vi "rsidr_core_global.vi"() -> ()   [LabVIEW 2020, in "Rohde&Schwarz RTx Oscilloscopes.lvlib"] (continued)
"Descriptive Name"="Start Power Safe Operating Area Measurement", "Data Type"=4, "Command"="POW:SOA:EXEC", "Access"=1, "Range Table"="", "Read Callback"="", "Write Callback"="", "Supported Models"="RTM|RTA", "Instrument Options"="", "Flags"=0, "Help"="Starts the safe operating area measurement.\n\nAvailable Repeated Capabilities:\nNone\n\nRemote-control command(s):\nPOWer:SOA:EXECute"}, {"Level"=3, "Class Only"=FALSE, "Identifier"="RSRTX_ATTR_RESTART_POWER_SAFE_OPERATING_AREA_MEASUREMENT", "Descriptive Name"="Restart Power Safe Operating Area Measurement", "Data Type"=4, "Command"="POW:SOA:REST", "Access"=1, "Range Table"="", "Read Callback"="", "Write Callback"="", "Supported Models"="RTM|RTA", "Instrument Options"="", "Flags"=0, "Help"="Restarts the measurement.\n\nAvailable Repeated Capabilities:\nNone\n\nRemote-control command(s):\nPOWer:SOA:RESTart"}, {"Level"=3, "Class Only"=FALSE, "Identifier"="RSRTX_ATTR_POWER_SAFE_OPERATING_AREA_ADD_REPORT", "Descriptive Name"="Power Safe Operating Area Add Report", "Data Type"=4, "Command"="POW:SOA:REP:ADD", "Access"=1, "Range Table"="", "Read Callback"="", "Write Callback"="", "Supported Models"="RTM|RTA", "Instrument Options"="", "Flags"=1, "Help"="Adds the result to the report list.\n\nAvailable Repeated Capabilities:\nNone\n\nRemote-control command(s):\nPOWer:SOA:REPort:ADD"}, {"Level"=3, "Class Only"=FALSE, "Identifier"="RSRTX_ATTR_POWER_SAFE_OPERATING_AREA_SCALE", "Descriptive Name"="Power Safe Operating Area Scale", "Data Type"=0, "Command"="POW:SOA:SCAL", "Access"=2, "Range Table"="rsrtx_rngScaleLinLog", "Read Callback"="", "Write Callback"="", "Supported Models"="RTM|RTA", "Instrument Options"="", "Flags"=0, "Help"="Sets the scale for the measurement.\n\nAvailable Repeated Capabilities:\nNone\n\nRemote-control command(s):\nPOWer:SOA:SCALe"}, {"Level"=3, "Class Only"=FALSE, "Identifier"="RSRTX_ATTR_POWER_SAFE_OPERATING_AREA_MASK_SCALE", "Descriptive Name"="Power Safe Operating Area Mask Scale", "Data Type"=0, "Command"="POW:SOA:SCAL:MASK", "Access"=2, "Range Table"="rsrtx_rngScaleLinLog", "Read Callback"="", "Write Callback"="", "Supported Models"="RTM|RTA", "Instrument Options"="", "Flags"=0, "Help"="Sets the scale for the mask, linear or logarithmic.\n\nAvailable Repeated Capabilities:\nNone\n\nRemote-control command(s):\nPOWer:SOA:SCALe:MASK"}, {"Level"=3, "Class Only"=FALSE, "Identifier"="RSRTX_ATTR_POWER_SAFE_OPERATING_AREA_DISPLAY_SCALE", "Descriptive Name"="Power Safe Operating Area Display Scale", "Data Type"=0, "Command"="POW:SOA:SCAL:DISP", "Access"=2, "Range Table"="rsrtx_rngScaleLinLog", "Read Callback"="", "Write Callback"="", "Supported Models"="RTM|RTA", "Instrument Options"="", "Flags"=0, "Help"="Sets a linear or a logarithmic scaled for the displayed results.\n\nAvailable Repeated Capabilities:\nNone\n\nRemote-control command(s):\nPOWer:SOA:SCALe:DISPlay"}, {"Level"=3, "Class Only"=FALSE, "Identifier"="RSRTX_ATTR_POWER_SAFE_OPERATING_AREA_LIN_ADD", "Descriptive Name"="Power Safe Operating Area Linear Add", "Data Type"=4, "Command"="POW:SOA:LIN:ADD", "Access"=1, "Range Table"="", "Read Callback"="", "Write Callback"="", "Supported Models"="RTM|RTA", "Instrument Options"="", "Flags"=0, "Help"="Adds a point.\n\nAvailable Repeated Capabilities:\nNone\n\nRemote-control command(s):\nPOWer:SOA:LINear:ADD"}, {"Level"=3, "Class Only"=FALSE, "Identifier"="RSRTX_ATTR_POWER_SAFE_OPERATING_AREA_LINEAR_INSERT", "Descriptive Name"="Power Safe Operating Area Linear Insert", "Data Type"=0, "Command"="POW:SOA:LIN:INS", "Access"=1, "Range Table"="", "Read Callback"="", "Write Callback"="", "Supported Models"="RTM|RTA", "Instrument Options"="", "Flags"=0, "Help"="Inserts a point.\n\nAvailable Repeated Capabilities:\nNone\n\nRemote-control command(s):\nPOWer:SOA:LINear:INSert"}, {"Level"=3, "Class Only"=FALSE, "Identifier"="RSRTX_ATTR_POWER_SAFE_OPERATING_AREA_LINEAR_REMOVE", "Descriptive Name"="Power Safe Operating Area Linear Remove", "Data Type"=0, "Command"="POW:SOA:LIN:REM", "Access"=1, "Range Table"="", "Read Callback"="", "Write Callback"="", "Supported Models"="RTM|RTA", "Instrument Options"="", "Flags"=0, "Help"="Removes a point.\n\nAvailable Repeated Capabilities:\nNone\n\nRemote-control command(s):\nPOWer:SOA:LINear:REMove"}, {"Level"=3, "Class Only"=FALSE, "Identifier"="RSRTX_ATTR_POWER_SAFE_OPERATING_AREA_LINEAR_COUNT", "Descriptive Name"="Power Safe Operating Area Linear Count", "Data Type"=0, "Command"="POW:SOA:LIN:COUN?", "Access"=0, "Range Table"="", "Read Callback"="", "Write Callback"="", "Supported Models"="RTM|RTA", "Instrument Options"="", "Flags"=0, "Help"="Queries the number of points.\n\nAvailable Repeated Capabilities:\nNone\n\nRemote-control command(s):\nPOWer:SOA:LINear:COUNt?"}, {"Level"=3, "Class Only"=FALSE, "Identifier"="RSRTX_ATTR_POWER_SAFE_OPERATING_AREA_LOGARITHMIC_ADD", "Descriptive Name"="Power Safe Operating Area Logarithmic Add", "Data Type"=4, "Command"="POW:SOA:LOG:ADD", "Access"=1, "Range Table"="", "Read Callback"="", "Write Callback"="", "Supported Models"="RTM|RTA", "Instrument Options"="", "Flags"=0, "Help"="Adds a point.\n\nAvailable Repeated Capabilities:\nNone\n\nRemote-control command(s):\nPOWer:SOA:LOGarithmic:ADD"}, {"Level"=3, "Class Only"=FALSE, "Identifier"="RSRTX_ATTR_POWER_SAFE_OPERATING_AREA_LOGARITHMIC_INSERT", "Descriptive Name"="Power Safe Operating Area Logarithmic Insert", "Data Type"=0, "Command"="POW:SOA:LOG:INS", "Access"=1, "Range Table"="", "Read Callback"="", "Write Callback"="", "Supported Models"="RTM|RTA", "Instrument Options"="", "Flags"=0, "Help"="Inserts a point.\n\nAvailable Repeated Capabilities:\nNone\n\nRemote-control command(s):\nPOWer:SOA:LOGarithmic:INSert"}, {"Level"=3, "Class Only"=FALSE, "Identifier"="RSRTX_ATTR_POWER_SAFE_OPERATING_AREA_LOGARITHMIC_REMOVE", "Descriptive Name"="Power Safe Operating Area Logarithmic Remove", "Data Type"=0, "Command"="POW:SOA:LOG:REM", "Access"=1, "Range Table"="", "Read Callback"="", "Write Callback"="", "Supported Models"="RTM|RTA", "Instrument Options"="", "Flags"=0, "Help"="Removes a point.\n\nAvailable Repeated Capabilities:\nNone\n\nRemote-control command(s):\nPOWer:SOA:LOGarithmic:REMove"}, {"Level"=3, "Class Only"=FALSE, "Identifier"="RSRTX_ATTR_POWER_SAFE_OPERATING_AREA_LOGARITHMIC_COUNT", "Descriptive Name"="Power Safe Operating Area Logarithmic Count", "Data Type"=0, "Command"="POW:SOA:LOG:COUN?", "Access"=0, "Range Table"="", "Read Callback"="", "Write Callback"="", "Supported Models"="RTM|RTA", "Instrument Options"="", "Flags"=0, "Help"="Queries the number of points.\n\nAvailable Repeated Capabilities:\nNone\n\nRemote-control command(s):\nPOWer:SOA:LOGarithmic:COUNt?"}, {"Level"=3, "Class Only"=FALSE, "Identifier"="RSRTX_ATTR_POWER_SAFE_OPERATING_AREA_SELECTED_POINT", "Descriptive Name"="Power Safe Operating Area Selected Point", "Data Type"=0, "Command"="", "Access"=2, "Range Table"="", "Read Callback"="", "Write Callback"="", "Supported Models"="", "Instrument Options"="", "Flags"=0, "Help"="Sets selector repeated capability Point.\n\nAvailable Repeated Capabilities:\nNone\n\nRemote-control command(s):\n"}, {"Level"=3, "Class Only"=TRUE, "Identifier"="", "Descriptive Name"="Point", "Data Type"=0, "Command"="", "Access"=0, "Range Table"="", "Read Callback"="", "Write Callback"="", "Supported Models"="", "Instrument Options"="", "Flags"=0, "Help"="Class for Point repcap. Points is selected with attribute RSRTX_ATTR_POWER_SAFE_OPERATING_AREA_SELECTED_POINT."}, {"Level"=4, "Class Only"=FALSE, "Identifier"="RSRTX_ATTR_POWER_SAFE_OPERATING_AREA_LINEAR_POINT_VOLTAGE", "Descriptive Name"="Power Safe Operating Area Linear Point Voltage", "Data Type"=1, "Command"="POW:SOA:LIN:POIN<Point>:VOLT", "Access"=2, "Range Table"="", "Read Callback"="rsrtx_FormatSOAPointRepCapReal_ReadCallback.vi", "Write Callback"="rsrtx_FormatSOAPointRepCapReal_WriteCallback.vi", "Supported Models"="RTM|RTA", "Instrument Options"="", "Flags"=0, "Help"="Sets the voltage for the correponding point.\n\nAvailable Repeated Capabilities:\nNone\n\nRemote-control command(s):\nPOWer:SOA:LINear:POINt<m>:VOLTage"}, {"Level"=4, "Class Only"=FALSE, "Identifier"="RSRTX_ATTR_POWER_SAFE_OPERATING_AREA_LINEAR_POINT_CURRENT", "Descriptive Name"="Power Safe Operating Area Linear Point Current", "Data Type"=1, "Command"="POW:SOA:LIN:POIN<Point>:CURR", "Access"=2, "Range Table"="", "Read Callback"="rsrtx_FormatSOAPointRepCapReal_ReadCallback.vi", "Write Callback"="rsrtx_FormatSOAPointRepCapReal_WriteCallback.vi", "Supported Models"="RTM|RTA", "Instrument Options"="", "Flags"=0, "Help"="Sets the current for the correponding point.\n\nAvailable Repeated Capabilities:\nNone\n\nRemote-control command(s):\nPOWer:SOA:LINear:POINt<m>:CURRent"}, {"Level"=4, "Class Only"=FALSE, "Identifier"="RSRTX_ATTR_POWER_SAFE_OPERATING_AREA_LINEAR_POINT_CURRENT_MIN", "Descriptive Name"="Power Safe Operating Area Linear Point Current Min", "Data Type"=1, "Command"="POW:SOA:LIN:POIN<Point>:CURR:MIN", "Access"=2, "Range Table"="", "Read Callback"="rsrtx_FormatSOAPointRepCapReal_ReadCallback.vi", "Write Callback"="rsrtx_FormatSOAPointRepCapReal_WriteCallback.vi", "Supported Models"="RTM|RTA", "Instrument Options"="", "Flags"=0, "Help"="Sets the minimum current for the correponding point.\n\nAvailable Repeated Capabilities:\nNone\n\nRemote-control command(s):\nPOWer:SOA:LINear:POINt<m>:CURRent:MINimum"}, {"Level"=4, "Class Only"=FALSE, "Identifier"="RSRTX_ATTR_POWER_SAFE_OPERATING_AREA_LINEAR_POINT_CURRENT_MAX", "Descriptive Name"="Power Safe Operating Area Linear Point Current Max", "Data Type"=1, "Command"="POW:SOA:LIN:POIN<Point>:CURR:MAX", "Access"=2, "Range Table"="", "Read Callback"="rsrtx_FormatSOAPointRepCapReal_ReadCallback.vi", "Write Callback"="rsrtx_FormatSOAPointRepCapReal_WriteCallback.vi", "Supported Models"="RTM|RTA", "Instrument Options"="", "Flags"=0, "Help"="Sets the maximum current for the correponding point.\n\nAvailable Repeated Capabilities:\nNone\n\nRemote-control command(s):\nPOWer:SOA:LINear:POINt<m>:CURRent:MAXimum"}, {"Level"=4, "Class Only"=FALSE, "Identifier"="RSRTX_ATTR_POWER_SAFE_OPERATING_AREA_LOGARITHMIC_POINT_VOLTAGE", "Descriptive Name"="Power Safe Operating Area Logarithmic Point Voltage", "Data Type"=1, "Command"="POW:SOA:LOG:POIN<Point>:VOLT", "Access"=2, "Range Table"="", "Read Callback"="rsrtx_FormatSOAPointRepCapReal_ReadCallback.vi", "Write Callback"="rsrtx_FormatSOAPointRepCapReal_WriteCallback.vi", "Supported Models"="RTM|RTA", "Instrument Options"="", "Flags"=0, "Help"="Sets the voltage for the correponding point.\n\nAvailable Repeated Capabilities:\nNone\n\nRemote-control command(s):\nPOWer:SOA:LOGarithmic:POINt<m>:VOLTage"}, {"Level"=4, "Class Only"=FALSE, "Identifier"="RSRTX_ATTR_POWER_SAFE_OPERATING_AREA_LOGARITHMIC_POINT_CURRENT", "Descriptive Name"="Power Safe Operating Area Logarithmic Point Current", "Data Type"=1, "Command"="POW:SOA:LOG:POIN<Point>:CURR", "Access"=2, "Range Table"="", "Read Callback"="rsrtx_FormatSOAPointRepCapReal_ReadCallback.vi", "Write Callback"="rsrtx_FormatSOAPointRepCapReal_WriteCallback.vi", "Supported Models"="RTM|RTA", "Instrument Options"="", "Flags"=0, "Help"="Sets the current for the correponding point.\n\nAvailable Repeated Capabilities:\nNone\n\nRemote-control command(s):\nPOWer:SOA:LOGarithmic:POINt<m>:CURRent"}, {"Level"=4, "Class Only"=FALSE, "Identifier"="RSRTX_ATTR_POWER_SAFE_OPERATING_AREA_LOGARITHMIC_POINT_CURRENT_MIN", "Descriptive Name"="Power Safe Operating Area Logarithmic Point Current Min", "Data Type"=1, "Command"="POW:SOA:LOG:POIN<Point>:CURR:MIN", "Access"=2, "Range Table"="", "Read Callback"="rsrtx_FormatSOAPointRepCapReal_ReadCallback.vi", "Write Callback"="rsrtx_FormatSOAPointRepCapReal_WriteCallback.vi", "Supported Models"="RTM|RTA", "Instrument Options"="", "Flags"=0, "Help"="Sets the minimum current for the correponding point.\n\nAvailable Repeated Capabilities:\nNone\n\nRemote-control command(s):\nPOWer:SOA:LOGarithmic:POINt<m>:CURRent:MINimum"}, {"Level"=4, "Class Only"=FALSE, "Identifier"="RSRTX_ATTR_POWER_SAFE_OPERATING_AREA_LOGARITHMIC_POINT_CURRENT_MAX", "Descriptive Name"="Power Safe Operating Area Logarithmic Point Current Max", "Data Type"=1, "Command"="POW:SOA:LOG:POIN<Point>:CURR:MAX", "Access"=2, "Range Table"="", "Read Callback"="rsrtx_FormatSOAPointRepCapReal_ReadCallback.vi", "Write Callback"="rsrtx_FormatSOAPointRepCapReal_WriteCallback.vi", "Supported Models"="RTM|RTA", "Instrument Options"="", "Flags"=0, "Help"="Sets the maximum current for the correponding point.\n\nAvailable Repeated Capabilities:\nNone\n\nRemote-control command(s):\nPOWer:SOA:LOGarithmic:POINt<m>:CURRent:MAXimum"}, {"Level"=3, "Class Only"=TRUE, "Identifier"="", "Descriptive Name"="Results", "Data Type"=0, "Command"="", "Access"=0, "Range Table"="", "Read Callback"="", "Write Callback"="", "Supported Models"="", "Instrument Options"="", "Flags"=0, "Help"="The results of &quot;Safe Operating Area&quot; measurements."}, {"Level"=4, "Class Only"=TRUE, "Identifier"="", "Descriptive Name"="Acquisition", "Data Type"=0, "Command"="", "Access"=0, "Range Table"="", "Read Callback"="", "Write Callback"="", "Supported Models"="", "Instrument Options"="", "Flags"=0, "Help"="Acquisition results."}, {"Level"=5, "Class Only"=FALSE, "Identifier"="RSRTX_ATTR_POWER_SAFE_OPERATING_AREA_RESULT_ACQUISITION_TOLERANCE", "Descriptive Name"="Power Safe Operating Area Result Acquisition Tolerance", "Data Type"=1, "Command"="POW:SOA:RES:ACQ:TOL", "Access"=2, "Range Table"="", "Read Callback"="", "Write Callback"="", "Supported Models"="RTM|RTA", "Instrument Options"="", "Flags"=0, "Help"="Sets acquisition tolerance in percent.\n\nAvailable Repeated Capabilities:\nNone\n\nRemote-control command(s):\nPOWer:SOA:RESult:ACQuisition:TOLerance"}, {"Level"=5, "Class Only"=FALSE, "Identifier"="RSRTX_ATTR_POWER_SAFE_OPERATING_AREA_RESULT_ACQUISITION_PASSED_RESULTS", "Descriptive Name"="Power Safe Operating Area Result Acquisition Passed Results", "Data Type"=0, "Command"="POW:SOA:RES:ACQ:PASS?", "Access"=0, "Range Table"="", "Read Callback"="", "Write Callback"="", "Supported Models"="RTM|RTA", "Instrument Options"="", "Flags"=0, "Help"="Returns the number of passed points, i.e they are within the defined safe operating area.\n\nAvailable Repeated Capabilities:\nNone\n\nRemote-control command(s):\nPOWer:SOA:RESult:ACQuisition:PASSed?"}, {"Level"=5, "Class Only"=FALSE, "Identifier"="RSRTX_ATTR_POWER_SAFE_OPERATING_AREA_RESULT_ACQUISITION_FAILED_RESULTS", "Descriptive Name"="Power Safe Operating Area Result Acquisition Failed Results", "Data Type"=0, "Command"="POW:SOA:RES:ACQ:FAIL?", "Access"=0, "Range Table"="", "Read Callback"="", "Write Callback"="", "Supported Models"="RTM|RTA", "Instrument Options"="", "Flags"=0, "Help"="Returns the number of points that failed, i.e they are not within the defined safe operating area.\n\nAvailable Repeated Capabilities:\nNone\n\nRemote-control command(s):\nPOWer:SOA:RESult:ACQuisition:FAILed?"}, {"Level"=5, "Class Only"=FALSE, "Identifier"="RSRTX_ATTR_POWER_SAFE_OPERATING_AREA_RESULT_ACQUISITION_FAILED_RATE", "Descriptive Name"="Power Safe Operating Area Result Acquisition Failed Rate", "Data Type"=1, "Command"="POW:SOA:RES:ACQ:FRAT?", "Access"=0, "Range Table"="", "Read Callback"="", "Write Callback"="", "Supported Models"="RTM|RTA", "Instrument Options"="", "Flags"=0, "Help"="Returns the total point fail rate, i.e the ratio of point hits to the number of tested points for the current acquisition.\n\nAvailable Repeated Capabilities:\nNone\n\nRemote-control command(s):\nPOWer:SOA:RESult:ACQuisition:FRATe?"}, {"Level"=5, "Class Only"=FALSE, "Identifier"="RSRTX_ATTR_POWER_SAFE_OPERATING_AREA_RESULT_ACQUISITION_NUMBER_OF_POINTS", "Descriptive Name"="Power Safe Operating Area Result Acquisition Number Of Points", "Data Type"=0, "Command"="POW:SOA:RES:ACQ:POIN?", "Access"=0, "Range Table"="", "Read Callback"="", "Write Callback"="", "Supported Models"="RTM|RTA", "Instrument Options"="", "Flags"=0, "Help"="Returns the number of points, considered for the current acquisition.\n\nAvailable Repeated Capabilities:\nNone\n\nRemote-control command(s):\nPOWer:SOA:RESult:ACQuisition:POINts?"}, {"Level"=5, "Class Only"=FALSE, "Identifier"="RSRTX_ATTR_POWER_SAFE_OPERATING_AREA_RESULT_ACQUISITION_STATUS", "Descriptive Name"="Power Safe Operating Area Result Acquisition Status", "Data Type"=3, "Command"="POW:SOA:RES:ACQ:STAT?", "Access"=0, "Range Table"="", "Read Callback"="", "Write Callback"="", "Supported Models"="RTM|RTA", "Instrument Options"="", "Flags"=0, "Help"="Returns the result, passed or failed, of the current aqcuisition measurement.\n\nAvailable Repeated Capabilities:\nNone\n\nRemote-control command(s):\nPOWer:SOA:RESult:ACQuisition:STATe?"}, {"Level"=5, "Class Only"=FALSE, "Identifier"="RSRTX_ATTR_POWER_SAFE_OPERATING_AREA_RESULT_ACQUISITION_VIOLATION_COUNT", "Descriptive Name"="Power Safe Operating Area Result Acquisition Violation Count", "Data Type"=0, "Command"="POW:SOA:RES:ACQ:VCO?", "Access"=0, "Range Table"="", "Read Callback"="", "Write Callback"="", "Supported Models"="RTM|RTA", "Instrument Options"="", "Flags"=0, "Help"="Returns the acquisition violation count.\n\nAvailable Repeated Capabilities:\nNone\n\nRemote-control command(s):\nPOWer:SOA:RESult:ACQuisition:VCOunt?"}, {"Level"=5, "Class Only"=TRUE, "Identifier"="", "Descriptive Name"="Point", "Data Type"=0, "Command"="", "Access"=0, "Range Table"="", "Read Callback"="", "Write Callback"="", "Supported Models"="", "Instrument Options"="", "Flags"=0, "Help"="Class for Point repcap. Points is selected with attribute RSRTX_ATTR_POWER_SAFE_OPERATING_AREA_SELECTED_POINT."}, {"Level"=6, "Class Only"=FALSE, "Identifier"="RSRTX_ATTR_POWER_SAFE_OPERATING_AREA_RESULT_ACQUISITION_VIOLATION", "Descriptive Name"="Power Safe Operating Area Result Acquisition Violation", "Data Type"=2, "Command"="POW:SOA:RES:ACQ:VIOL<Point>?", "Access"=0, "Range Table"="", "Read Callback"="rsrtx_FormatSOAPointRepCapString_ReadCallback.vi", "Write Callback"="", "Supported Models"="", "Instrument Options"="", "Flags"=0, "Help"="Returns the current and voltage value for the corresponding acquisition violation.\n\nAvailable Repeated Capabilities:\nNone\n\nRemote-control command(s):\nPOWer:SOA:RESult:ACQuisition:VIOLation<n>?"}, {"Level"=6, "Class Only"=FALSE, "Identifier"="RSRTX_ATTR_POWER_SAFE_OPERATING_AREA_RESULT_ACQUISITION_VIOLATION_CURRENT", "Descriptive Name"="Power Safe Operating Area Result Acquisition Violation Current", "Data Type"=1, "Command"="POW:SOA:RES:ACQ:VIOL<Point>:CURR?", "Access"=0, "Range Table"="", "Read Callback"="rsrtx_FormatSOAPointRepCapReal_ReadCallback.vi", "Write Callback"="", "Supported Models"="RTM|RTA", "Instrument Options"="", "Flags"=0, "Help"="Returns the current value for the corresponding acquisition violation point.\n\nAvailable Repeated Capabilities:\nNone\n\nRemote-control command(s):\nPOWer:SOA:RESult:ACQuisition:VIOLation<n>:CURRent?"}, {"Level"=6, "Class Only"=FALSE, "Identifier"="RSRTX_ATTR_POWER_SAFE_OPERATING_AREA_RESULT_ACQUISITION_VIOLATION_VOLTAGE", "Descriptive Name"="Power Safe Operating Area Result Acquisition Violation Voltage", "Data Type"=1, "Command"="POW:SOA:RES:ACQ:VIOL<Point>:VOLT?", "Access"=0, "Range Table"="", "Read Callback"="rsrtx_FormatSOAPointRepCapReal_ReadCallback.vi", "Write Callback"="", "Supported Models"="RTM|RTA", "Instrument Options"="", "Flags"=0, "Help"="Returns the voltage value for the corresponding acquisition violation point.\n\nAvailable Repeated Capabilities:\nNone\n\nRemote-control command(s):\nPOWer:SOA:RESult:ACQuisition:VIOLation<n>:VOLTage?"}, {"Level"=6, "Class Only"=TRUE, "Identifier"="", "Descriptive Name"="Voltage Data", "Data Type"=0, "Command"="", "Access"=0, "Range Table"="", "Read Callback"="", "Write Callback"="", "Supported Models"="", "Instrument Options"="", "Flags"=0, "Help"="Acquires voltage data."}, {"Level"=6, "Class Only"=TRUE, "Identifier"="", "Descriptive Name"="Voltage Data Conversion", "Data Type"=0, "Command"="", "Access"=0, "Range Table"="", "Read Callback"="", "Write Callback"="", "Supported Models"="", "Instrument Options"="", "Flags"=0, "Help"="Attributes for conversion of voltage data."}, {"Level"=7, "Class Only"=FALSE, "Identifier"="RSRTX_ATTR_POWER_SAFE_OPERATING_AREA_RESULT_ACQUISITION_VOLTAGE_DATA_CONVERSION_X_START", "Descriptive Name"="Power Safe Operating Area Result Acquisition Voltage Data Conversion X Start", "Data Type"=1, "Command"="POW:SOA:RES:ACQ:VIOL<Point>:VOLT:DATA:XOR?", "Access"=0, "Range Table"="", "Read Callback"="rsrtx_FormatSOAPointRepCapReal_ReadCallback.vi", "Write Callback"="", "Supported Models"="RTM|RTA", "Instrument Options"="", "Flags"=0, "Help"="Return the time of the first sample of the indicated waveform.\n\nAvailable Repeated Capabilities:\nNone\n\nRemote-control command(s):\nPOWer:SOA:RESult:ACQuisition:VIOLation<n>:VOLTage:DATA:XORigin?"}, {"Level"=7, "Class Only"=FALSE, "Identifier"="RSRTX_ATTR_POWER_SAFE_OPERATING_AREA_RESULT_ACQUISITION_VOLTAGE_DATA_CONVERSION_X_INCREMENT", "Descriptive Name"="Power Safe Operating Area Result Acquisition Voltage Data Conversion X Increment", "Data Type"=1, "Command"="POW:SOA:RES:ACQ:VIOL<Point>:VOLT:DATA:XINC?", "Access"=0, "Range Table"="", "Read Callback"="rsrtx_FormatSOAPointRepCapReal_ReadCallback.vi", "Write Callback"="", "Supported Models"="RTM|RTA", "Instrument Options"="", "Flags"=0, "Help"="Return the time difference between two adjacent samples of the indicated waveform.\n\nAvailable Repeated Capabilities:\nNone\n\nRemote-control command(s):\nPOWer:SOA:RESult:ACQuisition:VIOLation<n>:VOLTage:DATA:XINCrement?"}, {"Level"=7, "Class Only"=FALSE, "Identifier"="RSRTX_ATTR_POWER_SAFE_OPERATING_AREA_RESULT_ACQUISITION_VOLTAGE_DATA_CONVERSION_Y_START", "Descriptive Name"="Power Safe Operating Area Result Acquisition Voltage Data Conversion Y Start", "Data Type"=1, "Command"="POW:SOA:RES:ACQ:VIOL<Point>:VOLT:DATA:YOR?", "Access"=0, "Range Table"="", "Read Callback"="rsrtx_FormatSOAPointRepCapReal_ReadCallback.vi", "Write Callback"="", "Supported Models"="RTM|RTA", "Instrument Options"="", "Flags"=0, "Help"="Return the voltage value for binary value 0 of the indicated waveform.\n\nAvailable Repeated Capabilities:\nNone\n\nRemote-control command(s):\nPOWer:SOA:RESult:ACQuisition:VIOLation<n>:VOLTage:DATA:YORigin?"}, {"Level"=7, "Class Only"=FALSE, "Identifier"="RSRTX_ATTR_POWER_SAFE_OPERATING_AREA_RESULT_ACQUISITION_VOLTAGE_DATA_CONVERSION_Y_INCREMENT", "Descriptive Name"="Power Safe Operating Area Result Acquisition Voltage Data Conversion Y Increment", "Data Type"=1, "Command"="POW:SOA:RES:ACQ:VIOL<Point>:VOLT:DATA:YINC?", "Access"=0, "Range Table"="", "Read Callback"="rsrtx_FormatSOAPointRepCapReal_ReadCallback.vi", "Write Callback"="", "Supported Models"="RTM|RTA", "Instrument Options"="", "Flags"=0, "Help"="Return the voltage value per bit of the indicated waveform.\n\nAvailable Repeated Capabilities:\nNone\n\nRemote-control command(s):\nPOWer:SOA:RESult:ACQuisition:VIOLation<n>:VOLTage:DATA:YINCrement?"}, {"Level"=7, "Class Only"=FALSE, "Identifier"="RSRTX_ATTR_POWER_SAFE_OPERATING_AREA_RESULT_ACQUISITION_VOLTAGE_DATA_CONVERSION_Y_RESOLUTION", "Descriptive Name"="Power Safe Operating Area Result Acquisition Voltage Data Conversion Y Resolution", "Data Type"=0, "Command"="POW:SOA:RES:ACQ:VIOL<Point>:VOLT:DATA:YRES?", "Access"=0, "Range Table"="", "Read Callback"="rsrtx_FormatSOAPointRepCapInt_ReadCallback.vi", "Write Callback"="", "Supported Models"="RTM|RTA", "Instrument Options"="", "Flags"=0, "Help"="Return the vertical bit resolution of the indicated waveform.\n\nAvailable Repeated Capabilities:\nNone\n\nRemote-control command(s):\nPOWer:SOA:RESult:ACQuisition:VIOLation<n>:VOLTage:DATA:YRESolution?"}, {"Level"=6, "Class Only"=TRUE, "Identifier"="", "Descriptive Name"="Current Data", "Data Type"=0, "Command"="", "Access"=0, "Range Table"="", "Read Callback"="", "Write Callback"="", "Supported Models"="", "Instrument Options"="", "Flags"=0, "Help"="Acquires current data."}, {"Level"=6, "Class Only"=TRUE, "Identifier"="", "Descriptive Name"="Current Data Conversion", "Data Type"=0, "Command"="", "Access"=0, "Range Table"="", "Read Callback"="", "Write Callback"="", "Supported Models"="", "Instrument Options"="", "Flags"=0, "Help"="Attributes for conversion of current data."}, {"Level"=7, "Class Only"=FALSE, "Identifier"="RSRTX_ATTR_POWER_SAFE_OPERATING_AREA_RESULT_ACQUISITION_CURRENT_DATA_CONVERSION_X_START", "Descriptive Name"="Power Safe Operating Area Result Acquisition Current Data Conversion X Start", "Data Type"=1, "Command"="POW:SOA:RES:ACQ:VIOL<Point>:CURR:DATA:XOR?", "Access"=0, "Range Table"="", "Read Callback"="rsrtx_FormatSOAPointRepCapReal_ReadCallback.vi", "Write Callback"="", "Supported Models"="RTM|RTA", "Instrument Options"="", "Flags"=0, "Help"="Return the time of the first sample of the indicated waveform.\n\nAvailable Repeated Capabilities:\nNone\n\nRemote-control command(s):\nPOWer:SOA:RESult:ACQuisition:VIOLation<n>:CURRent:DATA:XORigin?"}, {"Level"=7, "Class Only"=FALSE, "Identifier"="RSRTX_ATTR_POWER_SAFE_OPERATING_AREA_RESULT_ACQUISITION_CURRENT_DATA_CONVERSION_X_INCREMENT", "Descriptive Name"="Power Safe Operating Area Result Acquisition Current Data Conversion X Increment", "Data Type"=1, "Command"="POW:SOA:RES:ACQ:VIOL<Point>:CURR:DATA:XINC?", "Access"=0, "Range Table"="", "Read Callback"="rsrtx_FormatSOAPointRepCapReal_ReadCallback.vi", "Write Callback"="", "Supported Models"="RTM|RTA", "Instrument Options"="", "Flags"=0, "Help"="Return the time difference between two adjacent samples of the indicated waveform.\n\nAvailable Repeated Capabilities:\nNone\n\nRemote-control command(s):\nPOWer:SOA:RESult:ACQuisition:VIOLation<n>:CURRent:DATA:XINCrement?"}, {"Level"=7, "Class Only"=FALSE, "Identifier"="RSRTX_ATTR_POWER_SAFE_OPERATING_AREA_RESULT_ACQUISITION_CURRENT_DATA_CONVERSION_Y_START", "Descriptive Name"="Power Safe Operating Area Result Acquisition Current Data Conversion Y Start", "Data Type"=1, "Command"="POW:SOA:RES:ACQ:VIOL<Point>:CURR:DATA:YOR?", "Access"=0, "Range Table"="", "Read Callback"="rsrtx_FormatSOAPointRepCapReal_ReadCallback.vi", "Write Callback"="", "Supported Models"="RTM|RTA", "Instrument Options"="", "Flags"=0, "Help"="Return the voltage value for binary value 0 of the indicated waveform.\n\nAvailable Repeated Capabilities:\nNone\n\nRemote-control command(s):\nPOWer:SOA:RESult:ACQuisition:VIOLation<n>:CURRent:DATA:YORigin?"}, {"Level"=7, "Class Only"=FALSE, "Identifier"="RSRTX_ATTR_POWER_SAFE_OPERATING_AREA_RESULT_ACQUISITION_CURRENT_DATA_CONVERSION_Y_INCREMENT", "Descriptive Name"="Power Safe Operating Area Result Acquisition Current Data Conversion Y Increment", "Data Type"=1, "Command"="POW:SOA:RES:ACQ:VIOL<Point>:CURR:DATA:YINC?", "Access"=0, "Range Table"="", "Read Callback"="rsrtx_FormatSOAPointRepCapReal_ReadCallback.vi", "Write Callback"="", "Supported Models"="RTM|RTA", "Instrument Options"="", "Flags"=0, "Help"="Return the voltage value per bit of the indicated waveform.\n\nAvailable Repeated Capabilities:\nNone\n\nRemote-control command(s):\nPOWer:SOA:RESult:ACQuisition:VIOLation<n>:CURRent:DATA:YINCrement?"}, {"Level"=7, "Class Only"=FALSE, "Identifier"="RSRTX_ATTR_POWER_SAFE_OPERATING_AREA_RESULT_ACQUISITION_CURRENT_DATA_CONVERSION_Y_RESOLUTION", "Descriptive Name"="Power Safe Operating Area Result Acquisition Current Data Conversion Y Resolution", "Data Type"=0, "Command"="POW:SOA:RES:ACQ:VIOL<Point>:CURR:DATA:YRES?", "Access"=0, "Range Table"="", "Read Callback"="rsrtx_FormatSOAPointRepCapInt_ReadCallback.vi", "Write Callback"="", "Supported Models"="RTM|RTA", "Instrument Options"="", "Flags"=0, "Help"="Return the vertical bit resolution of the indicated waveform.\n\nAvailable Repeated Capabilities:\nNone\n\nRemote-control command(s):\nPOWer:SOA:RESult:ACQuisition:VIOLation<n>:CURRent:DATA:YRESolution?"}, {"Level"=4, "Class Only"=TRUE, "Identifier"="", "Descriptive Name"="Total", "Data Type"=0, "Command"="", "Access"=0, "Range Table"="", "Read Callback"="", "Write Callback"="", "Supported Models"="", "Instrument Options"="", "Flags"=0, "Help"="Total results."}, {"Level"=5, "Class Only"=FALSE, "Identifier"="RSRTX_ATTR_POWER_SAFE_OPERATING_AREA_RESULT_TOTAL_TOLERANCE", "Descriptive Name"="Power Safe Operating Area Result Total Tolerance", "Data Type"=1, "Command"="POW:SOA:RES:TOT:TOL", "Access"=2, "Range Table"="", "Read Callback"="", "Write Callback"="", "Supported Models"="RTM|RTA", "Instrument Options"="", "Flags"=0, "Help"="Sets total tolerance in percent.\n\nAvailable Repeated Capabilities:\nNone\n\nRemote-control command(s):\nPOWer:SOA:RESult:TOTal:TOLerance"}, {"Level"=5, "Class Only"=FALSE, "Identifier"="RSRTX_ATTR_POWER_SAFE_OPERATING_AREA_RESULT_TOTAL_PASSED_RESULTS", "Descriptive Name"="Power Safe Operating Area Result Total Passed Results", "Data Type"=0, "Command"="POW:SOA:RES:TOT:PASS?", "Access"=0, "Range Table"="", "Read Callback"="", "Write Callback"="", "Supported Models"="RTM|RTA", "Instrument Options"="", "Flags"=0, "Help"="Returns the number of passed acquisitions, i.e they are within the defined safe operating area.\n\nAvailable Repeated Capabilities:\nNone\n\nRemote-control command(s):\nPOWer:SOA:RESult:TOTal:PASSed?"}, {"Level"=5, "Class Only"=FALSE, "Identifier"="RSRTX_ATTR_POWER_SAFE_OPERATING_AREA_RESULT_TOTAL_FAILED_RESULTS", "Descriptive Name"="Power Safe Operating Area Result Total Failed Results", "Data Type"=0, "Command"="POW:SOA:RES:TOT:FAIL?", "Access"=0, "Range Table"="", "Read Callback"="", "Write Callback"="", "Supported Models"="RTM|RTA", "Instrument Options"="", "Flags"=0, "Help"="Returns the total number of failed acquisitions, i.e they are not within the defined safe operating area.\n\nAvailable Repeated Capabilities:\nNone\n\nRemote-control command(s):\nPOWer:SOA:RESult:TOTal:FAILed?"}, {"Level"=5, "Class Only"=FALSE, "Identifier"="RSRTX_ATTR_POWER_SAFE_OPERATING_AREA_RESULT_TOTAL_FAILED_RATE", "Descriptive Name"="Power Safe Operating Area Result Total Failed Rate", "Data Type"=1, "Command"="POW:SOA:RES:TOT:FRAT?", "Access"=0, "Range Table"="", "Read Callback"="", "Write Callback"="", "Supported Models"="RTM|RTA", "Instrument Options"="", "Flags"=0, "Help"="Returns the total acquisition fail rate, i.e the ratio of acquisition hits to the number of tested acquisitions.\n\nAvailable Repeated Capabilities:\nNone\n\nRemote-control command(s):\nPOWer:SOA:RESult:TOTal:FRATe?"}, {"Level"=5, "Class Only"=FALSE, "Identifier"="RSRTX_ATTR_POWER_SAFE_OPERATING_AREA_RESULT_TOTAL_NUMBER_OF_ACQUISITIONS", "Descriptive Name"="Power Safe Operating Area Result Total Number Of Acquisitions", "Data Type"=0, "Command"="POW:SOA:RES:TOT:COUN?", "Access"=0, "Range Table"="", "Read Callback"="", "Write Callback"="", "Supported Models"="RTM|RTA", "Instrument Options"="", "Flags"=0, "Help"="Returns the total number of acquisitions used to determine the total result.\n\nAvailable Repeated Capabilities:\nNone\n\nRemote-control command(s):\nPOWer:SOA:RESult:TOTal:COUNt?"}, {"Level"=5, "Class Only"=FALSE, "Identifier"="RSRTX_ATTR_POWER_SAFE_OPERATING_AREA_RESULT_TOTAL_STATUS", "Descriptive Name"="Power Safe Operating Area Result Total Status", "Data Type"=3, "Command"="POW:SOA:RES:TOT:STAT?", "Access"=0, "Range Table"="", "Read Callback"="", "Write Callback"="", "Supported Models"="RTM|RTA", "Instrument Options"="", "Flags"=0, "Help"="Returns the result, passed or failed, of the total measurement.\n\nAvailable Repeated Capabilities:\nNone\n\nRemote-control command(s):\nPOWer:SOA:RESult:TOTal:STATe?"}, {"Level"=5, "Class Only"=FALSE, "Identifier"="RSRTX_ATTR_POWER_SAFE_OPERATING_AREA_RESULT_TOTAL_VIOLATION_COUNT", "Descriptive Name"="Power Safe Operating Area Result Total Violation Count", "Data Type"=0, "Command"="POW:SOA:RES:TOT:VCO?", "Access"=0, "Range Table"="", "Read Callback"="", "Write Callback"="", "Supported Models"="RTM|RTA", "Instrument Options"="", "Flags"=0, "Help"="Returns the total violation count.\n\nAvailable Repeated Capabilities:\nNone\n\nRemote-control command(s):\nPOWer:SOA:RESult:TOTal:VCOunt?"}, {"Level"=5, "Class Only"=FALSE, "Identifier"="RSRTX_ATTR_POWER_SAFE_OPERATING_AREA_RESULT_TOTAL_PASSED_SAMPLES", "Descriptive Name"="Power Safe Operating Area Result Total Passed Samples", "Data Type"=0, "Command"="POW:SOA:RES:TOT:SAMP:PASS?", "Access"=0, "Range Table"="", "Read Callback"="", "Write Callback"="", "Supported Models"="RTM|RTA", "Instrument Options"="", "Flags"=0, "Help"="Returns the number of passed samples, i.e they are within the defined safe operating area.\n\nAvailable Repeated Capabilities:\nNone\n\nRemote-control command(s):\nPOWer:SOA:RESult:TOTal:SAMPle:PASSed?"}, {"Level"=5, "Class Only"=FALSE, "Identifier"="RSRTX_ATTR_POWER_SAFE_OPERATING_AREA_RESULT_TOTAL_FAILED_SAMPLES", "Descriptive Name"="Power Safe Operating Area Result Total Failed Samples", "Data Type"=0, "Command"="POW:SOA:RES:TOT:SAMP:FAIL?", "Access"=0, "Range Table"="", "Read Callback"="", "Write Callback"="", "Supported Models"="RTM|RTA", "Instrument Options"="", "Flags"=0, "Help"="Returns the total number of failed samples, i.e they are not within the defined safe operating area.\n\nAvailable Repeated Capabilities:\nNone\n\nRemote-control command(s):\nPOWer:SOA:RESult:TOTal:SAMPle:FAILed?"}, {"Level"=5, "Class Only"=FALSE, "Identifier"="RSRTX_ATTR_POWER_SAFE_OPERATING_AREA_RESULT_TOTAL_NUMBER_OF_SAMPLES", "Descriptive Name"="Power Safe Operating Area Result Total Number Of Samples", "Data Type"=0, "Command"="POW:SOA:RES:TOT:SAMP:COUN?", "Access"=0, "Range Table"="", "Read Callback"="", "Write Callback"="", "Supported Models"="RTM|RTA", "Instrument Options"="", "Flags"=0, "Help"="Returns the total number of acquisitions used to determine the total result.\n\nAvailable Repeated Capabilities:\nNone\n\nRemote-control command(s):\nPOWer:SOA:RESult:TOTal:SAMPle:COUNt?"}, {"Level"=5, "Class Only"=TRUE, "Identifier"="", "Descriptive Name"="Point", "Data Type"=0, "Command"="", "Access"=0, "Range Table"="", "Read Callback"="", "Write Callback"="", "Supported Models"="", "Instrument Options"="", "Flags"=0, "Help"="Class for Point repcap. Points is selected with attribute RSRTX_ATTR_POWER_SAFE_OPERATING_AREA_SELECTED_POINT."}, {"Level"=6, "Class Only"=FALSE, "Identifier"="RSRTX_ATTR_POWER_SAFE_OPERATING_AREA_RESULT_TOTAL_VIOLATION", "Descriptive Name"="Power Safe Operating Area Result Total Violation", "Data Type"=2, "Command"="POW:SOA:RES:TOT:VIOL<Point>?", "Access"=0, "Range Table"="", "Read Callback"="rsrtx_FormatSOAPointRepCapString_ReadCallback.vi", "Write Callback"="", "Supported Models"="", "Instrument Options"="", "Flags"=0, "Help"="Returns the current and voltage value for the corresponding total violation.\n\nAvailable Repeated Capabilities:\nNone\n\nRemote-control command(s):\nPOWer:SOA:RESult:TOTal:VIOLation<n>?"}, {"Level"=6, "Class Only"=FALSE, "Identifier"="RSRTX_ATTR_POWER_SAFE_OPERATING_AREA_RESULT_TOTAL_VIOLATION_CURRENT", "Descriptive Name"="Power Safe Operating Area Result Total Violation Current", "Data Type"=1, "Command"="POW:SOA:RES:TOT:VIOL<Point>:CURR?", "Access"=0, "Range Table"="", "Read Callback"="rsrtx_FormatSOAPointRepCapReal_ReadCallback.vi", "Write Callback"="", "Supported Models"="RTM|RTA", "Instrument Options"="", "Flags"=0, "Help"="Returns the current of the total violation.\n\nAvailable Repeated Capabilities:\nNone\n\nRemote-control command(s):\nPOWer:SOA:RESult:TOTal:VIOLation<n>:CURRent?"}, {"Level"=6, "Class Only"=FALSE, "Identifier"="RSRTX_ATTR_POWER_SAFE_OPERATING_AREA_RESULT_TOTAL_VIOLATION_VOLTAGE", "Descriptive Name"="Power Safe Operating Area Result Total Violation Voltage", "Data Type"=1, "Command"="POW:SOA:RES:TOT:VIOL<Point>:VOLT?", "Access"=0, "Range Table"="", "Read Callback"="rsrtx_FormatSOAPointRepCapReal_ReadCallback.vi", "Write Callback"="", "Supported Models"="RTM|RTA", "Instrument Options"="", "Flags"=0, "Help"="Returns the voltage of the total violation.\n\nAvailable Repeated Capabilities:\nNone\n\nRemote-control command(s):\nPOWer:SOA:RESult:TOTal:VIOLation<n>:VOLTage?"}, {"Level"=6, "Class Only"=TRUE, "Identifier"="", "Descriptive Name"="Voltage Data", "Data Type"=0, "Command"="", "Access"=0, "Range Table"="", "Read Callback"="", "Write Callback"="", "Supported Models"="", "Instrument Options"="", "Flags"=0, "Help"="Acquires voltage data."}, {"Level"=6, "Class Only"=TRUE, "Identifier"="", "Descriptive Name"="Voltage Data Conversion", "Data Type"=0, "Command"="", "Access"=0, "Range Table"="", "Read Callback"="", "Write Callback"="", "Supported Models"="", "Instrument Options"="", "Flags"=0, "Help"="Attributes for conversion of voltage data."}, {"Level"=7, "Class Only"=FALSE, "Identifier"="RSRTX_ATTR_POWER_SAFE_OPERATING_AREA_RESULT_TOTAL_VOLTAGE_DATA_CONVERSION_X_START", "Descriptive Name"="Power Safe Operating Area Result Total Voltage Data Conversion X Start", "Data Type"=1, "Command"="POW:SOA:RES:TOT:VIOL<Point>:VOLT:DATA:XOR?", "Access"=0, "Range Table"="", "Read Callback"="rsrtx_FormatSOAPointRepCapReal_ReadCallback.vi", "Write Callback"="", "Supported Models"="RTM|RTA", "Instrument Options"="", "Flags"=0, "Help"="Return the time of the first sample of the indicated waveform.\n\nAvailable Repeated Capabilities:\nNone\n\nRemote-control command(s):\nPOWer:SOA:RESult:TOTal:VIOLation<n>:VOLTage:DATA:XORigin?"}, {"Level"=7, "Class Only"=FALSE, "Identifier"="RSRTX_ATTR_POWER_SAFE_OPERATING_AREA_RESULT_TOTAL_VOLTAGE_DATA_CONVERSION_X_INCREMENT", "Descriptive Name"="Power Safe Operating Area Result Total Voltage Data Conversion X Increment", "Data Type"=1, "Command"="POW:SOA:RES:TOT:VIOL<Point>:VOLT:DATA:XINC?", "Access"=0, "Range Table"="", "Read Callback"="rsrtx_FormatSOAPointRepCapReal_ReadCallback.vi", "Write Callback"="", "Supported Models"="RTM|RTA", "Instrument Options"="", "Flags"=0, "Help"="Return the time difference between two adjacent samples of the indicated waveform.\n\nAvailable Repeated Capabilities:\nNone\n\nRemote-control command(s):\nPOWer:SOA:RESult:TOTal:VIOLation<n>:VOLTage:DATA:XINCrement?"}, {"Level"=7, "Class Only"=FALSE, "Identifier"="RSRTX_ATTR_POWER_SAFE_OPERATING_AREA_RESULT_TOTAL_VOLTAGE_DATA_CONVERSION_Y_START", "Descriptive Name"="Power Safe Operating Area Result Total Voltage Data Conversion Y Start", "Data Type"=1, "Command"="POW:SOA:RES:TOT:VIOL<Point>:VOLT:DATA:YOR?", "Access"=0, "Range Table"="", "Read Callback"="rsrtx_FormatSOAPointRepCapReal_ReadCallback.vi", "Write Callback"="", "Supported Models"="RTM|RTA", "Instrument Options"="", "Flags"=0, "Help"="Return the voltage value for binary value 0 of the indicated waveform.\n\nAvailable Repeated Capabilities:\nNone\n\nRemote-control command(s):\nPOWer:SOA:RESult:TOTal:VIOLation<n>:VOLTage:DATA:YORigin?"}, {"Level"=7, "Class Only"=FALSE, "Identifier"="RSRTX_ATTR_POWER_SAFE_OPERATING_AREA_RESULT_TOTAL_VOLTAGE_DATA_CONVERSION_Y_INCREMENT", "Descriptive Name"="Power Safe Operating Area Result Total Voltage Data Conversion Y Increment", "Data Type"=1, "Command"="POW:SOA:RES:TOT:VIOL<Point>:VOLT:DATA:YINC?", "Access"=0, "Range Table"="", "Read Callback"="rsrtx_FormatSOAPointRepCapReal_ReadCallback.vi", "Write Callback"="", "Supported Models"="RTM|RTA", "Instrument Options"="", "Flags"=0, "Help"="Return the voltage value per bit of the indicated waveform.\n\nAvailable Repeated Capabilities:\nNone\n\nRemote-control command(s):\nPOWer:SOA:RESult:TOTal:VIOLation<n>:VOLTage:DATA:YINCrement?"}, {"Level"=7, "Class Only"=FALSE, "Identifier"="RSRTX_ATTR_POWER_SAFE_OPERATING_AREA_RESULT_TOTAL_VOLTAGE_DATA_CONVERSION_Y_RESOLUTION", "Descriptive Name"="Power Safe Operating Area Result Total Voltage Data Conversion Y Resolution", "Data Type"=0, "Command"="POW:SOA:RES:TOT:VIOL<Point>:VOLT:DATA:YRES?", "Access"=0, "Range Table"="", "Read Callback"="rsrtx_FormatSOAPointRepCapInt_ReadCallback.vi", "Write Callback"="", "Supported Models"="RTM|RTA", "Instrument Options"="", "Flags"=0, "Help"="Return the vertical bit resolution of 
